vi "test ByValRead.vi"(8 "error in (no error)":errorcluster, 11 "TestCase in":refnum<class "Interface Framework Single Object.lvclass">) -> (0 "error out":errorcluster, 3 "TestCase out":refnum<class "Interface Framework Single Object.lvclass">)   [LabVIEW 2009, in "Interface Framework Single Object.lvclass"]
uses:
  Interface Framework Single Object.lvclass
  Numeric Test Object/Interface Implementations/IIntByVal/IIntByVal.lvclass
  Interface Framework Single Object.lvclass/Interface Framework Single Object.ctl
  Numeric Test Object/Numeric Test Object.lvclass
  <vilib>/addons/_JKI Toolkits/VI Tester/TestCase.llb/TestCase.lvclass
  Source/Interfaceable Class/Interfaceable.lvclass
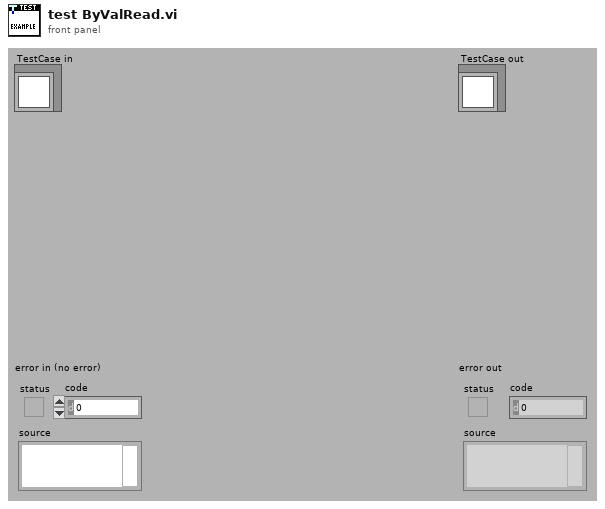
[diagram p1: front panel]
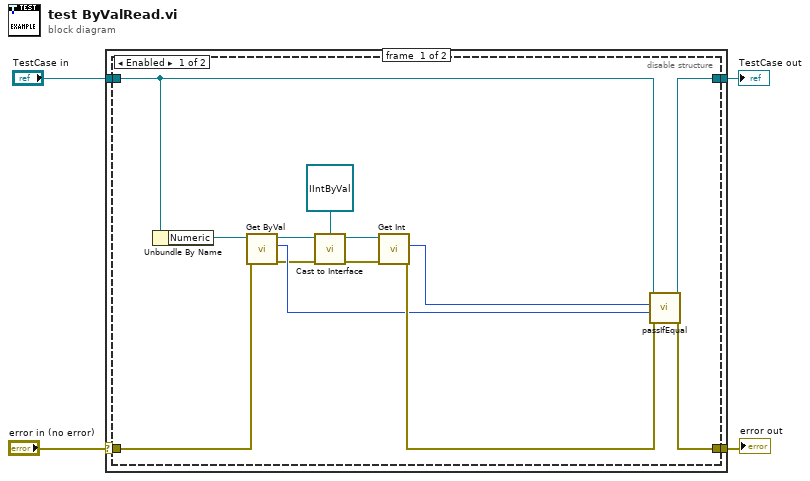
[diagram p0: block diagram]
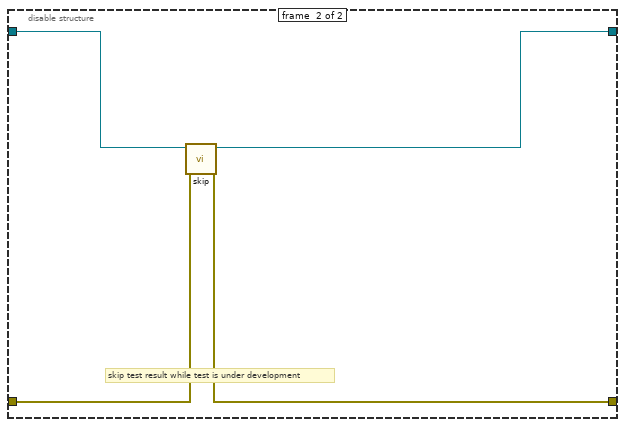
[diagram p2: hidden frame]
diagram:
  n1 = case shown="No Error" "error in (no error)" {
    selector: "error in (no error)" -> [w6 w27]
    tunnel: [w5 w27] -> w3
    tunnel: [w7 w26] -> w1
    tunnel: "TestCase in" -> [w8 w26]
    frame #0 {
      n2 = disable-structure shown="Enabled" {
        disable-tunnel: w8 -> [w19 w25]
        disable-tunnel: [w21 w22] -> w7
        disable-tunnel: w6 -> [w14 w24]
        disable-tunnel: [w20 w23] -> w5
        frame #0 {
          n3 = Unbundle By Name(w19) -> ("Numeric"=w17:refnum<class "Numeric Test Object.lvclass">)
          n4 = call-dynamic "Get ByVal.vi"("error in (no error)"=w14, "Numeric in"=w17) -> ("error out"=w10:errorcluster, "Int"=w12:i32, "Numeric out"=w16:refnum<class "Numeric Test Object.lvclass">)  [unwired: 7 in]
          n5 = call "Cast to Interface.vi"("Target Interface"=refnum<class "IIntByVal.lvclass"> refnum ("IIntByVal.lvclass"), "Interfaceable Object"=w16, "error in (no error)"=w10) -> ("Concrete Interface"=w15:refnum<class "IIntByVal.lvclass">, "error out"=w9:errorcluster)  [unwired: 5 in]
          n6 = call-dynamic "Get Int.vi"("error in (no error)"=w9, "IIntByVal in"=w15) -> ("error out"=w13:errorcluster, "Int"=w11:i32)  [unwired: 7 in, 1 out]
          n7 = call-dynamic "passIfEqual.vi"("error in (no error)"=w13, "y"=w12, "x"=w11, "TestCase in"=w19) -> ("error out"=w20:errorcluster, "TestCase out"=w21:refnum<class "Interface Framework Single Object.lvclass">)  [unwired: 6 in]
        }
        frame #1 {
          # "skip test result while test is under development"
          n8 = call <vilib>:"skip.vi"("error in (no error)"=w24, "TestCase in"=w25) -> ("error out"=w23:errorcluster, "TestCase out"=w22:refnum<class "Interface Framework Single Object.lvclass">)  [unwired: 8 in]
        }
      }
    }
    frame #1 {
    }
  }
  "error out" <- w3
  "TestCase out" <- w1
